vi "read record.vi"(8 "error in":errorcluster, 9 "timeout ms (-1)":i32=-1, 11 "connection":refnum<k5>) -> (0 "error out":errorcluster, 2 "data":string, 3 "header":T1, 4 "abort connection":bool)   [LabVIEW 2013]
uses:
  record header.ctl
  record types.ctl
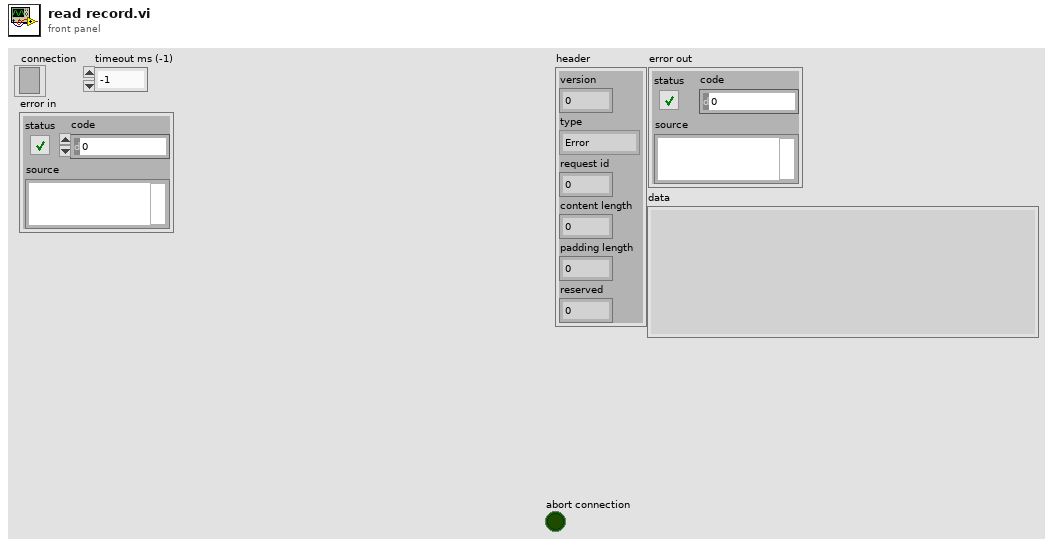
[diagram p1: front panel]
types:
  T1 = typedef "record header.ctl" = cluster{"version":u8, "type":T2, "request id":u16, "content length":u16, "padding length":u8, "reserved":u8}
  T2 = typedef "record types.ctl" = enum8{"Error", "Begin Request", "Abort Request", "End Request", "Parameters", "Standard Input", "Standard Output", "Standard Error", "Data", "Get Values", "Get Values Result", "Unknown Type"}
  T3 = enum16{"Standard", "Buffered", "CRLF", "Immediate"}
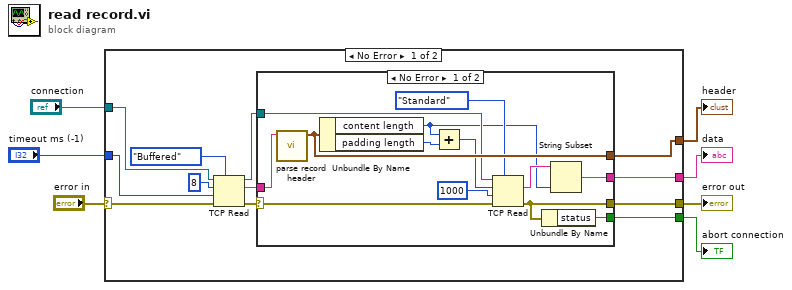
[diagram p0: block diagram]
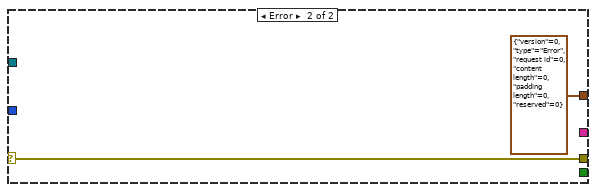
[diagram p3: hidden frame]
diagram:
  n1 = case shown="No Error" "error in" {
    selector: "error in" -> [w10 w35]
    tunnel: "connection" -> [w19 _]
    tunnel: "timeout ms (-1)" -> [w17 _]
    tunnel: [w14 T1 {"version"=0, "type"=enum."Error", "request id"=0, "content length"=0, "padding length"=0, "reserved"=0} ("header")] -> w5
    tunnel: [w12 w35] -> w4
    tunnel: [w11 _] -> w3
    tunnel: [w8 _] -> w1
    frame No Error {
      n2 = TCP Read(connection ID=w19, bytes to read=8, error in (no error)=w10, 7:T3."Buffered" ("mode (standard)"), 9:w17) -> (connection ID out=w13:refnum<k5>, data out=w15:string, error out=w9:errorcluster)
      n3 = case shown="No Error" w9 {
        selector: w9 -> [w24 w33]
        tunnel: w15 -> [w32 _]
        tunnel: [w31 _] -> w14
        tunnel: w13 -> [w26 _]
        tunnel: [w23 w33] -> w12
        tunnel: [w21 _] -> w11
        tunnel: [w22 _] -> w8
        frame No Error {
          n4 = call "parse record header.vi"("data"=w32) -> ("header"=w31:T1)  [unwired: 10 in]
          n5 = Unbundle By Name(w31) -> ("content length"=w20:u16, "padding length"=w30:u8)
          n6 = Add(x=w20, y=w30) -> (x+y=w29:u16)
          n7 = TCP Read(connection ID=w26, bytes to read=w29, error in (no error)=w24, 7:T3."Standard" ("mode (standard)"), 9:1000 ("timeout ms (25000)")) -> (data out=w25:string, error out=w23:errorcluster)  [unwired: 1 out]
          n8 = Unbundle By Name(w23) -> ("status"=w22:bool)
          n9 = String Subset(string=w25, length (rest)=w20) -> (substring=w21:string)  [unwired: 1 in]
        }
        frame Error {
        }
      }
    }
    frame Error {
    }
  }
  "header" <- w5
  "error out" <- w4
  "data" <- w3
  "abort connection" <- w1
